vi "Parameter Filter - By Label Decimal.vi"(2 "Label Decimal":i32, 7 "Parameters Array (in)":T1[](array[typedef])) -> (8 "Filtered Parameters Array (out)":T1[](array[typedef]))   [LabVIEW 2017] (continued)
"Channel Speed"=100, "Label Decimal"=117, "Label Name"="Label_165", "Min Rate (mS)"=720, "Max Rate (mS)"=1080, "SDI"=2, "SSM"=0, "Create SDI"=FALSE, "Create SSM"=FALSE, "Create Parity"=FALSE, "Parameter Name"="eng_rb2_lbl165_b10_28", "Start Bit"=10, "Number of Bits"=19, "Scale"="1", "Offset"="0", "Signed"=FALSE, "Unit"="N/A", "Encoding"=enum."Discrete", "Default Value"="0"}, {"Core Number"=0, "Channel Number"=23, "Channel Name"="ENG_RB2", "Channel Speed"=100, "Label Decimal"=119, "Label Name"="Label_167", "Min Rate (mS)"=720, "Max Rate (mS)"=1080, "SDI"=2, "SSM"=0, "Create SDI"=FALSE, "Create SSM"=FALSE, "Create Parity"=FALSE, "Parameter Name"="eng_rb2_lbl167_b10_28", "Start Bit"=10, "Number of Bits"=19, "Scale"="1", "Offset"="0", "Signed"=FALSE, "Unit"="N/A", "Encoding"=enum."Discrete", "Default Value"="0"}, {"Core Number"=0, "Channel Number"=23, "Channel Name"="ENG_RB2", "Channel Speed"=100, "Label Decimal"=120, "Label Name"="Label_170", "Min Rate (mS)"=720, "Max Rate (mS)"=1080, "SDI"=2, "SSM"=0, "Create SDI"=FALSE, "Create SSM"=FALSE, "Create Parity"=FALSE, "Parameter Name"="eng_rb2_lbl170_b10_28", "Start Bit"=10, "Number of Bits"=19, "Scale"="1", "Offset"="0", "Signed"=FALSE, "Unit"="N/A", "Encoding"=enum."Discrete", "Default Value"="0"}, {"Core Number"=0, "Channel Number"=23, "Channel Name"="ENG_RB2", "Channel Speed"=100, "Label Decimal"=125, "Label Name"="Label_175", "Min Rate (mS)"=720, "Max Rate (mS)"=1080, "SDI"=2, "SSM"=0, "Create SDI"=FALSE, "Create SSM"=FALSE, "Create Parity"=FALSE, "Parameter Name"="eng_rb2_lbl175_b10_28", "Start Bit"=10, "Number of Bits"=19, "Scale"="1", "Offset"="0", "Signed"=FALSE, "Unit"="N/A", "Encoding"=enum."Discrete", "Default Value"="0"}, {"Core Number"=0, "Channel Number"=23, "Channel Name"="ENG_RB2", "Channel Speed"=100, "Label Decimal"=126, "Label Name"="Label_176", "Min Rate (mS)"=720, "Max Rate (mS)"=1080, "SDI"=2, "SSM"=0, "Create SDI"=FALSE, "Create SSM"=FALSE, "Create Parity"=FALSE, "Parameter Name"="eng_rb2_lbl176_b10_28", "Start Bit"=10, "Number of Bits"=19, "Scale"="1", "Offset"="0", "Signed"=FALSE, "Unit"="N/A", "Encoding"=enum."Discrete", "Default Value"="0"}, {"Core Number"=0, "Channel Number"=23, "Channel Name"="ENG_RB2", "Channel Speed"=100, "Label Decimal"=127, "Label Name"="Label_177", "Min Rate (mS)"=720, "Max Rate (mS)"=1080, "SDI"=2, "SSM"=0, "Create SDI"=FALSE, "Create SSM"=FALSE, "Create Parity"=FALSE, "Parameter Name"="eng_rb2_lbl177_b10_28", "Start Bit"=10, "Number of Bits"=19, "Scale"="1", "Offset"="0", "Signed"=FALSE, "Unit"="N/A", "Encoding"=enum."Discrete", "Default Value"="0"}, {"Core Number"=0, "Channel Number"=23, "Channel Name"="ENG_RB2", "Channel Speed"=100, "Label Decimal"=129, "Label Name"="Label_201", "Min Rate (mS)"=720, "Max Rate (mS)"=1080, "SDI"=2, "SSM"=0, "Create SDI"=FALSE, "Create SSM"=FALSE, "Create Parity"=FALSE, "Parameter Name"="eng_rb2_lbl201_b10_28", "Start Bit"=10, "Number of Bits"=19, "Scale"="1", "Offset"="0", "Signed"=FALSE, "Unit"="N/A", "Encoding"=enum."Discrete", "Default Value"="0"}, {"Core Number"=0, "Channel Number"=23, "Channel Name"="ENG_RB2", "Channel Speed"=100, "Label Decimal"=130, "Label Name"="Label_202", "Min Rate (mS)"=720, "Max Rate (mS)"=1080, "SDI"=2, "SSM"=0, "Create SDI"=FALSE, "Create SSM"=FALSE, "Create Parity"=FALSE, "Parameter Name"="eng_rb2_lbl202_b10_28", "Start Bit"=10, "Number of Bits"=19, "Scale"="1", "Offset"="0", "Signed"=FALSE, "Unit"="N/A", "Encoding"=enum."Discrete", "Default Value"="0"}, {"Core Number"=0, "Channel Number"=23, "Channel Name"="ENG_RB2", "Channel Speed"=100, "Label Decimal"=132, "Label Name"="Label_204", "Min Rate (mS)"=720, "Max Rate (mS)"=1080, "SDI"=2, "SSM"=0, "Create SDI"=FALSE, "Create SSM"=FALSE, "Create Parity"=FALSE, "Parameter Name"="eng_rb2_lbl204_b10_28", "Start Bit"=10, "Number of Bits"=19, "Scale"="1", "Offset"="0", "Signed"=FALSE, "Unit"="N/A", "Encoding"=enum."Discrete", "Default Value"="0"}, {"Core Number"=0, "Channel Number"=23, "Channel Name"="ENG_RB2", "Channel Speed"=100, "Label Decimal"=139, "Label Name"="Label_213", "Min Rate (mS)"=800, "Max Rate (mS)"=1200, "SDI"=2, "SSM"=0, "Create SDI"=FALSE, "Create SSM"=FALSE, "Create Parity"=FALSE, "Parameter Name"="eng_rb2_lbl213_b10_28", "Start Bit"=10, "Number of Bits"=19, "Scale"="1", "Offset"="0", "Signed"=FALSE, "Unit"="N/A", "Encoding"=enum."Discrete", "Default Value"="0"}, {"Core Number"=0, "Channel Number"=23, "Channel Name"="ENG_RB2", "Channel Speed"=100, "Label Decimal"=64, "Label Name"="Label_100", "Min Rate (mS)"=800, "Max Rate (mS)"=1200, "SDI"=2, "SSM"=0, "Create SDI"=FALSE, "Create SSM"=FALSE, "Create Parity"=FALSE, "Parameter Name"="eng_rb2_lbl100_b13_27", "Start Bit"=13, "Number of Bits"=15, "Scale"="1", "Offset"="0", "Signed"=FALSE, "Unit"="N/A", "Encoding"=enum."Discrete", "Default Value"="0"}, {"Core Number"=0, "Channel Number"=23, "Channel Name"="ENG_RB2", "Channel Speed"=100, "Label Decimal"=66, "Label Name"="Label_102", "Min Rate (mS)"=800, "Max Rate (mS)"=1200, "SDI"=2, "SSM"=0, "Create SDI"=FALSE, "Create SSM"=FALSE, "Create Parity"=FALSE, "Parameter Name"="eng_rb2_lbl102_b13_27", "Start Bit"=13, "Number of Bits"=15, "Scale"="1", "Offset"="0", "Signed"=FALSE, "Unit"="N/A", "Encoding"=enum."Discrete", "Default Value"="0"}, {"Core Number"=0, "Channel Number"=1, "Channel Name"="RDC20_ENG_LA1", "Channel Speed"=100, "Label Decimal"=213, "Label Name"="Label_325", "Min Rate (mS)"=40, "Max Rate (mS)"=60, "SDI"=0, "SSM"=3, "Create SDI"=FALSE, "Create SSM"=FALSE, "Create Parity"=FALSE, "Parameter Name"="rdc20_eng_la1_lbl325_b10_28", "Start Bit"=10, "Number of Bits"=19, "Scale"="0.0006866", "Offset"="0", "Signed"=TRUE, "Unit"="Degrees", "Encoding"=enum."BNR", "Default Value"="0"}, {"Core Number"=0, "Channel Number"=1, "Channel Name"="RDC20_ENG_LA1", "Channel Speed"=100, "Label Decimal"=91, "Label Name"="Label_133", "Min Rate (mS)"=40, "Max Rate (mS)"=60, "SDI"=0, "SSM"=3, "Create SDI"=FALSE, "Create SSM"=FALSE, "Create Parity"=FALSE, "Parameter Name"="rdc20_eng_la1_lbl133_b10_28", "Start Bit"=10, "Number of Bits"=19, "Scale"="0.0006866", "Offset"="0", "Signed"=TRUE, "Unit"="Degrees", "Encoding"=enum."BNR", "Default Value"="0"}, {"Core Number"=0, "Channel Number"=1, "Channel Name"="RDC20_ENG_LA1", "Channel Speed"=100, "Label Decimal"=104, "Label Name"="Label_150", "Min Rate (mS)"=800, "Max Rate (mS)"=1200, "SDI"=0, "SSM"=3, "Create SDI"=FALSE, "Create SSM"=FALSE, "Create Parity"=FALSE, "Parameter Name"="rdc20_eng_la1_lbl150_b11_27", "Start Bit"=11, "Number of Bits"=17, "Scale"="1", "Offset"="0", "Signed"=FALSE, "Unit"="hh.mm.ss", "Encoding"=enum."BNR", "Default Value"="0"}, {"Core Number"=0, "Channel Number"=1, "Channel Name"="RDC20_ENG_LA1", "Channel Speed"=100, "Label Decimal"=39, "Label Name"="Label_47", "Min Rate (mS)"=800, "Max Rate (mS)"=1200, "SDI"=0, "SSM"=3, "Create SDI"=FALSE, "Create SSM"=FALSE, "Create Parity"=FALSE, "Parameter Name"="rdc20_eng_la1_lbl47_b10_27", "Start Bit"=10, "Number of Bits"=18, "Scale"="1", "Offset"="0", "Signed"=FALSE, "Unit"="N/A", "Encoding"=enum."BNR", "Default Value"="0"}, {"Core Number"=0, "Channel Number"=1, "Channel Name"="RDC20_ENG_LA1", "Channel Speed"=100, "Label Decimal"=188, "Label Name"="Label_274", "Min Rate (mS)"=800, "Max Rate (mS)"=1200, "SDI"=0, "SSM"=3, "Create SDI"=FALSE, "Create SSM"=FALSE, "Create Parity"=FALSE, "Parameter Name"="rdc20_eng_la1_lbl274_b18_28", "Start Bit"=18, "Number of Bits"=11, "Scale"="0.5", "Offset"="0", "Signed"=TRUE, "Unit"="Deg C", "Encoding"=enum."BNR", "Default Value"="0"}, {"Core Number"=0, "Channel Number"=1, "Channel Name"="RDC20_ENG_LA1", "Channel Speed"=100, "Label Decimal"=189, "Label Name"="Label_275", "Min Rate (mS)"=800, "Max Rate (mS)"=1200, "SDI"=0, "SSM"=3, "Create SDI"=FALSE, "Create SSM"=FALSE, "Create Parity"=FALSE, "Parameter Name"="rdc20_eng_la1_lbl275_b18_28", "Start Bit"=18, "Number of Bits"=11, "Scale"="0.5", "Offset"="0", "Signed"=TRUE, "Unit"="Deg C", "Encoding"=enum."BNR", "Default Value"="0"}, {"Core Number"=0, "Channel Number"=1, "Channel Name"="RDC20_ENG_LA1", "Channel Speed"=100, "Label Decimal"=184, "Label Name"="Label_270", "Min Rate (mS)"=80, "Max Rate (mS)"=120, "SDI"=0, "SSM"=0, "Create SDI"=FALSE, "Create SSM"=FALSE, "Create Parity"=FALSE, "Parameter Name"="rdc20_eng_la1_lbl270_b10_28", "Start Bit"=10, "Number of Bits"=19, "Scale"="1", "Offset"="0", "Signed"=FALSE, "Unit"="N/A", "Encoding"=enum."Discrete", "Default Value"="0"}, {"Core Number"=0, "Channel Number"=1, "Channel Name"="RDC20_ENG_LA1", "Channel Speed"=100, "Label Decimal"=185, "Label Name"="Label_271", "Min Rate (mS)"=80, "Max Rate (mS)"=120, "SDI"=0, "SSM"=0, "Create SDI"=FALSE, "Create SSM"=FALSE, "Create Parity"=FALSE, "Parameter Name"="rdc20_eng_la1_lbl271_b10_28", "Start Bit"=10, "Number of Bits"=19, "Scale"="1", "Offset"="0", "Signed"=FALSE, "Unit"="N/A", "Encoding"=enum."Discrete", "Default Value"="0"}, {"Core Number"=0, "Channel Number"=1, "Channel Name"="RDC20_ENG_LA1", "Channel Speed"=100, "Label Decimal"=186, "Label Name"="Label_272", "Min Rate (mS)"=80, "Max Rate (mS)"=120, "SDI"=0, "SSM"=0, "Create SDI"=FALSE, "Create SSM"=FALSE, "Create Parity"=FALSE, "Parameter Name"="rdc20_eng_la1_lbl272_b10_28", "Start Bit"=10, "Number of Bits"=19, "Scale"="1", "Offset"="0", "Signed"=FALSE, "Unit"="N/A", "Encoding"=enum."Discrete", "Default Value"="0"}, {"Core Number"=0, "Channel Number"=1, "Channel Name"="RDC20_ENG_LA1", "Channel Speed"=100, "Label Decimal"=187, "Label Name"="Label_273", "Min Rate (mS)"=80, "Max Rate (mS)"=120, "SDI"=0, "SSM"=0, "Create SDI"=FALSE, "Create SSM"=FALSE, "Create Parity"=FALSE, "Parameter Name"="rdc20_eng_la1_lbl273_b10_28", "Start Bit"=10, "Number of Bits"=19, "Scale"="1", "Offset"="0", "Signed"=FALSE, "Unit"="N/A", "Encoding"=enum."Discrete", "Default Value"="0"}, {"Core Number"=0, "Channel Number"=1, "Channel Name"="RDC20_ENG_LA1", "Channel Speed"=100, "Label Decimal"=151, "Label Name"="Label_227", "Min Rate (mS)"=80, "Max Rate (mS)"=120, "SDI"=0, "SSM"=0, "Create SDI"=FALSE, "Create SSM"=FALSE, "Create Parity"=FALSE, "Parameter Name"="rdc20_eng_la1_lbl227_b10_28", "Start Bit"=10, "Number of Bits"=19, "Scale"="1", "Offset"="0", "Signed"=FALSE, "Unit"="N/A", "Encoding"=enum."Discrete", "Default Value"="0"}, {"Core Number"=0, "Channel Number"=1, "Channel Name"="RDC20_ENG_LA1", "Channel Speed"=100, "Label Decimal"=105, "Label Name"="Label_151", "Min Rate (mS)"=800, "Max Rate (mS)"=1200, "SDI"=0, "SSM"=0, "Create SDI"=FALSE, "Create SSM"=FALSE, "Create Parity"=FALSE, "Parameter Name"="rdc20_eng_la1_lbl151_b10_27", "Start Bit"=10, "Number of Bits"=18, "Scale"="1", "Offset"="0", "Signed"=FALSE, "Unit"="N/A", "Encoding"=enum."Discrete", "Default Value"="0"}, {"Core Number"=0, "Channel Number"=2, "Channel Name"="RDC20_ENG_LA2", "Channel Speed"=100, "Label Decimal"=213, "Label Name"="Label_325", "Min Rate (mS)"=40, "Max Rate (mS)"=60, "SDI"=0, "SSM"=3, "Create SDI"=FALSE, "Create SSM"=FALSE, "Create Parity"=FALSE, "Parameter Name"="rdc20_eng_la2_lbl325_b10_28", "Start Bit"=10, "Number of Bits"=19, "Scale"="0.0006866", "Offset"="0", "Signed"=TRUE, "Unit"="Degrees", "Encoding"=enum."BNR", "Default Value"="0"}, {"Core Number"=0, "Channel Number"=2, "Channel Name"="RDC20_ENG_LA2", "Channel Speed"=100, "Label Decimal"=91, "Label Name"="Label_133", "Min Rate (mS)"=40, "Max Rate (mS)"=60, "SDI"=0, "SSM"=3, "Create SDI"=FALSE, "Create SSM"=FALSE, "Create Parity"=FALSE, "Parameter Name"="rdc20_eng_la2_lbl133_b10_28", "Start Bit"=10, "Number of Bits"=19, "Scale"="0.0006866", "Offset"="0", "Signed"=TRUE, "Unit"="Degrees", "Encoding"=enum."BNR", "Default Value"="0"}, {"Core Number"=0, "Channel Number"=2, "Channel Name"="RDC20_ENG_LA2", "Channel Speed"=100, "Label Decimal"=104, "Label Name"="Label_150", "Min Rate (mS)"=800, "Max Rate (mS)"=1200, "SDI"=0, "SSM"=3, "Create SDI"=FALSE, "Create SSM"=FALSE, "Create Parity"=FALSE, "Parameter Name"="rdc20_eng_la2_lbl150_b11_27", "Start Bit"=11, "Number of Bits"=17, "Scale"="1", "Offset"="0", "Signed"=FALSE, "Unit"="hh.mm.ss", "Encoding"=enum."BNR", "Default Value"="0"}, {"Core Number"=0, "Channel Number"=2, "Channel Name"="RDC20_ENG_LA2", "Channel Speed"=100, "Label Decimal"=39, "Label Name"="Label_47", "Min Rate (mS)"=800, "Max Rate (mS)"=1200, "SDI"=0, "SSM"=3, "Create SDI"=FALSE, "Create SSM"=FALSE, "Create Parity"=FALSE, "Parameter Name"="rdc20_eng_la2_lbl47_b10_27", "Start Bit"=10, "Number of Bits"=18, "Scale"="1", "Offset"="0", "Signed"=FALSE, "Unit"="N/A", "Encoding"=enum."BNR", "Default Value"="0"}, {"Core Number"=0, "Channel Number"=2, "Channel Name"="RDC20_ENG_LA2", "Channel Speed"=100, "Label Decimal"=188, "Label Name"="Label_274", "Min Rate (mS)"=800, "Max Rate (mS)"=1200, "SDI"=0, "SSM"=3, "Create SDI"=FALSE, "Create SSM"=FALSE, "Create Parity"=FALSE, "Parameter Name"="rdc20_eng_la2_lbl274_b18_28", "Start Bit"=18, "Number of Bits"=11, "Scale"="0.5", "Offset"="0", "Signed"=TRUE, "Unit"="Deg C", "Encoding"=enum."BNR", "Default Value"="0"}, {"Core Number"=0, "Channel Number"=2, "Channel Name"="RDC20_ENG_LA2", "Channel Speed"=100, "Label Decimal"=189, "Label Name"="Label_275", "Min Rate (mS)"=800, "Max Rate (mS)"=1200, "SDI"=0, "SSM"=3, "Create SDI"=FALSE, "Create SSM"=FALSE, "Create Parity"=FALSE, "Parameter Name"="rdc20_eng_la2_lbl275_b18_28", "Start Bit"=18, "Number of Bits"=11, "Scale"="0.5", "Offset"="0", "Signed"=TRUE, "Unit"="Deg C", "Encoding"=enum."BNR", "Default Value"="0"}, {"Core Number"=0, "Channel Number"=2, "Channel Name"="RDC20_ENG_LA2", "Channel Speed"=100, "Label Decimal"=184, "Label Name"="Label_270", "Min Rate (mS)"=80, "Max Rate (mS)"=120, "SDI"=0, "SSM"=0, "Create SDI"=FALSE, "Create SSM"=FALSE, "Create Parity"=FALSE, "Parameter Name"="rdc20_eng_la2_lbl270_b10_28", "Start Bit"=10, "Number of Bits"=19, "Scale"="1", "Offset"="0", "Signed"=FALSE, "Unit"="N/A", "Encoding"=enum."Discrete", "Default Value"="0"}, {"Core Number"=0, "Channel Number"=2, "Channel Name"="RDC20_ENG_LA2", "Channel Speed"=100, "Label Decimal"=185, "Label Name"="Label_271", "Min Rate (mS)"=80, "Max Rate (mS)"=120, "SDI"=0, "SSM"=0, "Create SDI"=FALSE, "Create SSM"=FALSE, "Create Parity"=FALSE, "Parameter Name"="rdc20_eng_la2_lbl271_b10_28", "Start Bit"=10, "Number of Bits"=19, "Scale"="1", "Offset"="0", "Signed"=FALSE, "Unit"="N/A", "Encoding"=enum."Discrete", "Default Value"="0"}, {"Core Number"=0, "Channel Number"=2, "Channel Name"="RDC20_ENG_LA2", "Channel Speed"=100, "Label Decimal"=186, "Label Name"="Label_272", "Min Rate (mS)"=80, "Max Rate (mS)"=120, "SDI"=0, "SSM"=0, "Create SDI"=FALSE, "Create SSM"=FALSE, "Create Parity"=FALSE, "Parameter Name"="rdc20_eng_la2_lbl272_b10_28", "Start Bit"=10, "Number of Bits"=19, "Scale"="1", "Offset"="0", "Signed"=FALSE, "Unit"="N/A", "Encoding"=enum."Discrete", "Default Value"="0"}, {"Core Number"=0, "Channel Number"=2, "Channel Name"="RDC20_ENG_LA2", "Channel Speed"=100, "Label Decimal"=187, "Label Name"="Label_273", "Min Rate (mS)"=80, "Max Rate (mS)"=120, "SDI"=0, "SSM"=0, "Create SDI"=FALSE, "Create SSM"=FALSE, "Create Parity"=FALSE, "Parameter Name"="rdc20_eng_la2_lbl273_b10_28", "Start Bit"=10, "Number of Bits"=19, "Scale"="1", "Offset"="0", "Signed"=FALSE, "Unit"="N/A", "Encoding"=enum."Discrete", "Default Value"="0"}, {"Core Number"=0, "Channel Number"=2, "Channel Name"="RDC20_ENG_LA2", "Channel Speed"=100, "Label Decimal"=151, "Label Name"="Label_227", "Min Rate (mS)"=80, "Max Rate (mS)"=120, "SDI"=0, "SSM"=0, "Create SDI"=FALSE, "Create SSM"=FALSE, "Create Parity"=FALSE, "Parameter Name"="rdc20_eng_la2_lbl227_b10_28", "Start Bit"=10, "Number of Bits"=19, "Scale"="1", "Offset"="0", "Signed"=FALSE, "Unit"="N/A", "Encoding"=enum."Discrete", "Default Value"="0"}, {"Core Number"=0, "Channel Number"=2, "Channel Name"="RDC20_ENG_LA2", "Channel Speed"=100, "Label Decimal"=105, "Label Name"="Label_151", "Min Rate (mS)"=800, "Max Rate (mS)"=1200, "SDI"=0, "SSM"=0, "Create SDI"=FALSE, "Create SSM"=FALSE, "Create Parity"=FALSE, "Parameter Name"="rdc20_eng_la2_lbl151_b10_27", "Start Bit"=10, "Number of Bits"=18, "Scale"="1", "Offset"="0", "Signed"=FALSE, "Unit"="N/A", "Encoding"=enum."Discrete", "Default Value"="0"}, {"Core Number"=0, "Channel Number"=3, "Channel Name"="RDC17_ENG_LB1", "Channel Speed"=100, "Label Decimal"=213, "Label Name"="Label_325", "Min Rate (mS)"=40, "Max Rate (mS)"=60, "SDI"=1, "SSM"=3, "Create SDI"=FALSE, "Create SSM"=FALSE, "Create Parity"=FALSE, "Parameter Name"="rdc17_eng_lb1_lbl325_b10_28", "Start Bit"=10, "Number of Bits"=19, "Scale"="0.0006866", "Offset"="0", "Signed"=TRUE, "Unit"="Degrees", "Encoding"=enum."BNR", "Default Value"="0"}, {"Core Number"=0, "Channel Number"=3, "Channel Name"="RDC17_ENG_LB1", "Channel Speed"=100, "Label Decimal"=91, "Label Name"="Label_133", "Min Rate (mS)"=40, "Max Rate (mS)"=60, "SDI"=1, "SSM"=3, "Create SDI"=FALSE, "Create SSM"=FALSE, "Create Parity"=FALSE, "Parameter Name"="rdc17_eng_lb1_lbl133_b10_28", "Start Bit"=10, "Number of Bits"=19, "Scale"="0.0006866", "Offset"="0", "Signed"=TRUE, "Unit"="Degrees", "Encoding"=enum."BNR", "Default Value"="0"}, {"Core Number"=0, "Channel Number"=3, "Channel Name"="RDC17_ENG_LB1", "Channel Speed"=100, "Label Decimal"=104, "Label Name"="Label_150", "Min Rate (mS)"=800, "Max Rate (mS)"=1200, "SDI"=1, "SSM"=3, "Create SDI"=FALSE, "Create SSM"=FALSE, "Create Parity"=FALSE, "Parameter Name"="rdc17_eng_lb1_lbl150_b11_27", "Start Bit"=11, "Number of Bits"=17, "Scale"="1", "Offset"="0", "Signed"=FALSE, "Unit"="hh.mm.ss", "Encoding"=enum."BNR", "Default Value"="0"}, {"Core Number"=0, "Channel Number"=3, "Channel Name"="RDC17_ENG_LB1", "Channel Speed"=100, "Label Decimal"=39, "Label Name"="Label_47", "Min Rate (mS)"=800, "Max Rate (mS)"=1200, "SDI"=1, "SSM"=3, "Create SDI"=FALSE, "Create SSM"=FALSE, "Create Parity"=FALSE, "Parameter Name"="rdc17_eng_lb1_lbl47_b10_27", "Start Bit"=10, "Number of Bits"=18, "Scale"="1", "Offset"="0", "Signed"=FALSE, "Unit"="N/A", "Encoding"=enum."BNR", "Default Value"="0"}, {"Core Number"=0, "Channel Number"=3, "Channel Name"="RDC17_ENG_LB1", "Channel Speed"=100, "Label Decimal"=188, "Label Name"="Label_274", "Min Rate (mS)"=800, "Max Rate (mS)"=1200, "SDI"=1, "SSM"=3, "Create SDI"=FALSE, "Create SSM"=FALSE, "Create Parity"=FALSE, "Parameter Name"="rdc17_eng_lb1_lbl274_b18_28", "Start Bit"=18, "Number of Bits"=11, "Scale"="0.5", "Offset"="0", "Signed"=TRUE, "Unit"="Deg C", "Encoding"=enum."BNR", "Default Value"="0"}, {"Core Number"=0, "Channel Number"=3, "Channel Name"="RDC17_ENG_LB1", "Channel Speed"=100, "Label Decimal"=189, "Label Name"="Label_275", "Min Rate (mS)"=800, "Max Rate (mS)"=1200, "SDI"=1, "SSM"=3, "Create SDI"=FALSE, "Create SSM"=FALSE, "Create Parity"=FALSE, "Parameter Name"="rdc17_eng_lb1_lbl275_b18_28", "Start Bit"=18, "Number of Bits"=11, "Scale"="0.5", "Offset"="0", "Signed"=TRUE, "Unit"="Deg C", "Encoding"=enum."BNR", "Default Value"="0"}, {"Core Number"=0, "Channel Number"=3, "Channel Name"="RDC17_ENG_LB1", "Channel Speed"=100, "Label Decimal"=184, "Label Name"="Label_270", "Min Rate (mS)"=80, "Max Rate (mS)"=120, "SDI"=1, "SSM"=0, "Create SDI"=FALSE, "Create SSM"=FALSE, "Create Parity"=FALSE, "Parameter Name"="rdc17_eng_lb1_lbl270_b10_28", "Start Bit"=10, "Number of Bits"=19, "Scale"="1", "Offset"="0", "Signed"=FALSE, "Unit"="N/A", "Encoding"=enum."Discrete", "Default Value"="0"}, {"Core Number"=0, "Channel Number"=3, "Channel Name"="RDC17_ENG_LB1", "Channel Speed"=100, "Label Decimal"=185, "Label Name"="Label_271", "Min Rate (mS)"=80, "Max Rate (mS)"=120, "SDI"=1, "SSM"=0, "Create SDI"=FALSE, "Create SSM"=FALSE, "Create Parity"=FALSE, "Parameter Name"="rdc17_eng_lb1_lbl271_b10_28", "Start Bit"=10, "Number of Bits"=19, "Scale"="1", "Offset"="0", "Signed"=FALSE, "Unit"="N/A", "Encoding"=enum."Discrete", "Default Value"="0"}, {"Core Number"=0, "Channel Number"=3, "Channel Name"="RDC17_ENG_LB1", "Channel Speed"=100, "Label Decimal"=186, "Label Name"="Label_272", "Min Rate (mS)"=80, "Max Rate (mS)"=120, "SDI"=1, "SSM"=0, "Create SDI"=FALSE, "Create SSM"=FALSE, "Create Parity"=FALSE, "Parameter Name"="rdc17_eng_lb1_lbl272_b10_28", "Start Bit"=10, "Number of Bits"=19, "Scale"="1", "Offset"="0", "Signed"=FALSE, "Unit"="N/A", "Encoding"=enum."Discrete", "Default Value"="0"}, {"Core Number"=0, "Channel Number"=3, "Channel Name"="RDC17_ENG_LB1", "Channel Speed"=100, "Label Decimal"=187, "Label Name"="Label_273", "Min Rate (mS)"=80, "Max Rate (mS)"=120, "SDI"=1, "SSM"=0, "Create SDI"=FALSE, "Create SSM"=FALSE, "Create Parity"=FALSE, "Parameter Name"="rdc17_eng_lb1_lbl273_b10_28", "Start Bit"=10, "Number of Bits"=19, "Scale"="1", "Offset"="0", "Signed"=FALSE, "Unit"="N/A", "Encoding"=enum."Discrete", "Default Value"="0"}, {"Core Number"=0, "Channel Number"=3, "Channel Name"="RDC17_ENG_LB1", "Channel Speed"=100, "Label Decimal"=151, "Label Name"="Label_227", "Min Rate (mS)"=80, "Max Rate (mS)"=120, "SDI"=1, "SSM"=0, "Create SDI"=FALSE, "Create SSM"=FALSE, "Create Parity"=FALSE, "Parameter Name"="rdc17_eng_lb1_lbl227_b10_28", "Start Bit"=10, "Number of Bits"=19, "Scale"="1", "Offset"="0", "Signed"=FALSE, "Unit"="N/A", "Encoding"=enum."Discrete", "Default Value"="0"}, {"Core Number"=0, "Channel Number"=3, "Channel Name"="RDC17_ENG_LB1", "Channel Speed"=100, "Label Decimal"=105, "Label Name"="Label_151", "Min Rate (mS)"=800, "Max Rate (mS)"=1200, "SDI"=1, "SSM"=0, "Create SDI"=FALSE, "Create SSM"=FALSE, "Create Parity"=FALSE, "Parameter Name"="rdc17_eng_lb1_lbl151_b10_27", "Start Bit"=10, "Number of Bits"=18, "Scale"="1", "Offset"="0", "Signed"=FALSE, "Unit"="N/A", "Encoding"=enum."Discrete", "Default Value"="0"}, {"Core Number"=0, "Channel Number"=4, "Channel Name"="RDC17_ENG_LB2", "Channel Speed"=100, "Label Decimal"=213, "Label Name"="Label_325", "Min Rate (mS)"=40, "Max Rate (mS)"=60, "SDI"=1, "SSM"=3, "Create SDI"=FALSE, "Create SSM"=FALSE, "Create Parity"=FALSE, "Parameter Name"="rdc17_eng_lb2_lbl325_b10_28", "Start Bit"=10, "Number of Bits"=19, "Scale"="0.0006866", "Offset"="0", "Signed"=TRUE, "Unit"="Degrees", "Encoding"=enum."BNR", "Default Value"="0"}, {"Core Number"=0, "Channel Number"=4, "Channel Name"="RDC17_ENG_LB2", "Channel Speed"=100, "Label Decimal"=91, "Label Name"="Label_133", "Min Rate (mS)"=40, "Max Rate (mS)"=60, "SDI"=1, "SSM"=3, "Create SDI"=FALSE, "Create SSM"=FALSE, "Create Parity"=FALSE, "Parameter Name"="rdc17_eng_lb2_lbl133_b10_28", "Start Bit"=10, "Number of Bits"=19, "Scale"="0.0006866", "Offset"="0", "Signed"=TRUE, "Unit"="Degrees", "Encoding"=enum."BNR", "Default Value"="0"}, {"Core Number"=0, "Channel Number"=4, "Channel Name"="RDC17_ENG_LB2", "Channel Speed"=100, "Label Decimal"=104, "Label Name"="Label_150", "Min Rate (mS)"=800, "Max Rate (mS)"=1200, "SDI"=1, "SSM"=3, "Create SDI"=FALSE, "Create SSM"=FALSE, "Create Parity"=FALSE, "Parameter Name"="rdc17_eng_lb2_lbl150_b11_27", "Start Bit"=11, "Number of Bits"=17, "Scale"="1", "Offset"="0", "Signed"=FALSE, "Unit"="hh.mm.ss", "Encoding"=enum."BNR", "Default Value"="0"}, {"Core Number"=0, "Channel Number"=4, "Channel Name"="RDC17_ENG_LB2", "Channel Speed"=100, "Label Decimal"=39, "Label Name"="Label_47", "Min Rate (mS)"=800, "Max Rate (mS)"=1200, "SDI"=1, "SSM"=3, "Create SDI"=FALSE, "Create SSM"=FALSE, "Create Parity"=FALSE, "Parameter Name"="rdc17_eng_lb2_lbl47_b10_27", "Start Bit"=10, "Number of Bits"=18, "Scale"="1", "Offset"="0", "Signed"=FALSE, "Unit"="N/A", "Encoding"=enum."BNR", "Default Value"="0"}, {"Core Number"=0, "Channel Number"=4, "Channel Name"="RDC17_ENG_LB2", "Channel Speed"=100, "Label Decimal"=188, "Label Name"="Label_274", "Min Rate (mS)"=800, "Max Rate (mS)"=1200, "SDI"=1, "SSM"=3, "Create SDI"=FALSE, "Create SSM"=FALSE, "Create Parity"=FALSE, "Parameter Name"="rdc17_eng_lb2_lbl274_b18_28", "Start Bit"=18, "Number of Bits"=11, "Scale"="0.5", "Offset"="0", "Signed"=TRUE, "Unit"="Deg C", "Encoding"=enum."BNR", "Default Value"="0"}, {"Core Number"=0, "Channel Number"=4, "Channel Name"="RDC17_ENG_LB2", "Channel Speed"=100, "Label Decimal"=189, "Label Name"="Label_275", "Min Rate (mS)"=800, "Max Rate (mS)"=1200, "SDI"=1, "SSM"=3, "Create SDI"=FALSE, "Create SSM"=FALSE, "Create Parity"=FALSE, "Parameter Name"="rdc17_eng_lb2_lbl275_b18_28", "Start Bit"=18, "Number of Bits"=11, "Scale"="0.5", "Offset"="0", "Signed"=TRUE, "Unit"="Deg C", "Encoding"=enum."BNR", "Default Value"="0"}, {"Core Number"=0, "Channel Number"=4, "Channel Name"="RDC17_ENG_LB2", "Channel Speed"=100, "Label Decimal"=184, "Label Name"="Label_270", "Min Rate (mS)"=80, "Max Rate (mS)"=120, "SDI"=1, "SSM"=0, "Create SDI"=FALSE, "Create SSM"=FALSE, "Create Parity"=FALSE, "Parameter Name"="rdc17_eng_lb2_lbl270_b10_28", "Start Bit"=10, "Number of Bits"=19, "Scale"="1", "Offset"="0", "Signed"=FALSE, "Unit"="N/A", "Encoding"=enum."Discrete", "Default Value"="0"}, {"Core Number"=0, "Channel Number"=4, "Channel Name"="RDC17_ENG_LB2", "Channel Speed"=100, "Label Decimal"=185, "Label Name"="Label_271", "Min Rate (mS)"=80, "Max Rate (mS)"=120, "SDI"=1, "SSM"=0, "Create SDI"=FALSE, "Create SSM"=FALSE, "Create Parity"=FALSE, "Parameter Name"="rdc17_eng_lb2_lbl271_b10_28", "Start Bit"=10, "Number of Bits"=19, "Scale"="1", "Offset"="0", "Signed"=FALSE, "Unit"="N/A", "Encoding"=enum."Discrete", "Default Value"="0"}, {"Core Number"=0, "Channel Number"=4, "Channel Name"="RDC17_ENG_LB2", "Channel Speed"=100, "Label Decimal"=186, "Label Name"="Label_272", "Min Rate (mS)"=80, "Max Rate (mS)"=120, "SDI"=1, "SSM"=0, "Create SDI"=FALSE, "Create SSM"=FALSE, "Create Parity"=FALSE, "Parameter Name"="rdc17_eng_lb2_lbl272_b10_28", "Start Bit"=10, "Number of Bits"=19, "Scale"="1", "Offset"="0", "Signed"=FALSE, "Unit"="N/A", "Encoding"=enum."Discrete", "Default Value"="0"}, {"Core Number"=0, "Channel Number"=4, "Channel Name"="RDC17_ENG_LB2", "Channel Speed"=100, "Label Decimal"=187, "Label Name"="Label_273", "Min Rate (mS)"=80, "Max Rate (mS)"=120, "SDI"=1, "SSM"=0, "Create SDI"=FALSE, "Create SSM"=FALSE, "Create Parity"=FALSE, "Parameter Name"="rdc17_eng_lb2_lbl273_b10_28", "Start Bit"=10, "Number of Bits"=19, "Scale"="1", "Offset"="0", "Signed"=FALSE, "Unit"="N/A", "Encoding"=enum."Discrete", "Default Value"="0"}, {"Core Number"=0, "Channel Number"=4, "Channel Name"="RDC17_ENG_LB2", "Channel Speed"=100, "Label Decimal"=151, "Label Name"="Label_227", "Min Rate (mS)"=80, "Max Rate (mS)"=120, "SDI"=1, "SSM"=0, "Create SDI"=FALSE, "Create SSM"=FALSE, "Create Parity"=FALSE, "Parameter Name"="rdc17_eng_lb2_lbl227_b10_28", "Start Bit"=10, "Number of Bits"=19, "Scale"="1", "Offset"="0", "Signed"=FALSE, "Unit"="N/A", "Encoding"=enum."Discrete", "Default Value"="0"}, {"Core Number"=0, "Channel Number"=4, "Channel Name"="RDC17_ENG_LB2", "Channel Speed"=100, "Label Decimal"=105, "Label Name"="Label_151", "Min Rate (mS)"=800, "Max Rate (mS)"=1200, "SDI"=1, "SSM"=0, "Create SDI"=FALSE, "Create SSM"=FALSE, "Create Parity"=FALSE, "Parameter Name"="rdc17_eng_lb2_lbl151_b10_27", "Start Bit"=10, "Number of Bits"=18, "Scale"="1", "Offset"="0", "Signed"=FALSE, "Unit"="N/A", "Encoding"=enum."Discrete", "Default Value"="0"}, {"Core Number"=0, "Channel Number"=5, "Channel Name"="RDC22_ENG_RA1", "Channel Speed"=100, "Label Decimal"=213, "Label Name"="Label_325", "Min Rate (mS)"=40, "Max Rate (mS)"=60, "SDI"=2, "SSM"=3, "Create SDI"=FALSE, "Create SSM"=FALSE, "Create Parity"=FALSE, "Parameter Name"="rdc22_eng_ra1_lbl325_b10_28", "Start Bit"=10, "Number of Bits"=19, "Scale"="0.0006866", "Offset"="0", "Signed"=TRUE, "Unit"="Degrees", "Encoding"=enum."BNR", "Default Value"="0"}, {"Core Number"=0, "Channel Number"=5, "Channel Name"="RDC22_ENG_RA1", "Channel Speed"=100, "Label Decimal"=91, "Label Name"="Label_133", "Min Rate (mS)"=40, "Max Rate (mS)"=60, "SDI"=2, "SSM"=3, "Create SDI"=FALSE, "Create SSM"=FALSE, "Create Parity"=FALSE, "Parameter Name"="rdc22_eng_ra1_lbl133_b10_28", "Start Bit"=10, "Number of Bits"=19, "Scale"="0.0006866", "Offset"="0", "Signed"=TRUE, "Unit"="Degrees", "Encoding"=enum."BNR", "Default Value"="0"}, {"Core Number"=0, "Channel Number"=5, "Channel Name"="RDC22_ENG_RA1", "Channel Speed"=100, "Label Decimal"=104, "Label Name"="Label_150", "Min Rate (mS)"=800, "Max Rate (mS)"=1200, "SDI"=2, "SSM"=3, "Create SDI"=FALSE, "Create SSM"=FALSE, "Create Parity"=FALSE, "Parameter Name"="rdc22_eng_ra1_lbl150_b11_27", "Start Bit"=11, "Number of Bits"=17, "Scale"="1", "Offset"="0", "Signed"=FALSE, "Unit"="hh.mm.ss", "Encoding"=enum."BNR", "Default Value"="0"}, {"Core Number"=0, "Channel Number"=5, "Channel Name"="RDC22_ENG_RA1", "Channel Speed"=100, "Label Decimal"=39, "Label Name"="Label_47", "Min Rate (mS)"=800, "Max Rate (mS)"=1200, "SDI"=2, "SSM"=3, "Create SDI"=FALSE, "Create SSM"=FALSE, "Create Parity"=FALSE, "Parameter Name"="rdc22_eng_ra1_lbl47_b10_27", "Start Bit"=10, "Number of Bits"=18, "Scale"="1", "Offset"="0", "Signed"=FALSE, "Unit"="N/A", "Encoding"=enum."BNR", "Default Value"="0"}, {"Core Number"=0, "Channel Number"=5, "Channel Name"="RDC22_ENG_RA1", "Channel Speed"=100, "Label Decimal"=188, "Label Name"="Label_274", "Min Rate (mS)"=800, "Max Rate (mS)"=1200, "SDI"=2, "SSM"=3, "Create SDI"=FALSE, "Create SSM"=FALSE, "Create Parity"=FALSE, "Parameter Name"="rdc22_eng_ra1_lbl274_b18_28", "Start Bit"=18, "Number of Bits"=11, "Scale"="0.5", "Offset"="0", "Signed"=TRUE, "Unit"="Deg C", "Encoding"=enum."BNR", "Default Value"="0"}, {"Core Number"=0, "Channel Number"=5, "Channel Name"="RDC22_ENG_RA1", "Channel Speed"=100, "Label Decimal"=189, "Label Name"="Label_275", "Min Rate (mS)"=800, "Max Rate (mS)"=1200, "SDI"=2, "SSM"=3, "Create SDI"=FALSE, "Create SSM"=FALSE, "Create Parity"=FALSE, "Parameter Name"="rdc22_eng_ra1_lbl275_b18_28", "Start Bit"=18, "Number of Bits"=11, "Scale"="0.5", "Offset"="0", "Signed"=TRUE, "Unit"="Deg C", "Encoding"=enum."BNR", "Default Value"="0"}, {"Core Number"=0, "Channel Number"=5, "Channel Name"="RDC22_ENG_RA1", "Channel Speed"=100, "Label Decimal"=184, "Label Name"="Label_270", "Min Rate (mS)"=80, "Max Rate (mS)"=120, "SDI"=2, "SSM"=0, "Create SDI"=FALSE, "Create SSM"=FALSE, "Create Parity"=FALSE, "Parameter Name"="rdc22_eng_ra1_lbl270_b10_28", "Start Bit"=10, "Number of Bits"=19, "Scale"="1", "Offset"="0", "Signed"=FALSE, "Unit"="N/A", "Encoding"=enum."Discrete", "Default Value"="0"}, {"Core Number"=0, "Channel Number"=5, "Channel Name"="RDC22_ENG_RA1", "Channel Speed"=100, "Label Decimal"=185, "Label Name"="Label_271", "Min Rate (mS)"=80, "Max Rate (mS)"=120, "SDI"=2, "SSM"=0, "Create SDI"=FALSE, "Create SSM"=FALSE, "Create Parity"=FALSE, "Parameter Name"="rdc22_eng_ra1_lbl271_b10_28", "Start Bit"=10, "Number of Bits"=19, "Scale"="1", "Offset"="0", "Signed"=FALSE, "Unit"="N/A", "Encoding"=enum."Discrete", "Default Value"="0"}, {"Core Number"=0, "Channel Number"=5, "Channel Name"="RDC22_ENG_RA1", "Channel Speed"=100, "Label Decimal"=186, "Label Name"="Label_272", "Min Rate (mS)"=80, "Max Rate (mS)"=120, "SDI"=2, "SSM"=0, "Create SDI"=FALSE, "Create SSM"=FALSE, "Create Parity"=FALSE, "Parameter Name"="rdc22_eng_ra1_lbl272_b10_28", "Start Bit"=10, "Number of Bits"=19, "Scale"="1", "Offset"="0", "Signed"=FALSE, "Unit"="N/A", "Encoding"=enum."Discrete", "Default Value"="0"}, {"Core Number"=0, "Channel Number"=5, "Channel Name"="RDC22_ENG_RA1", "Channel Speed"=100, "Label Decimal"=187, "Label Name"="Label_273", "Min Rate (mS)"=80, "Max Rate (mS)"=120, "SDI"=2, "SSM"=0, "Create SDI"=FALSE, "Create SSM"=FALSE, "Create Parity"=FALSE, "Parameter Name"="rdc22_eng_ra1_lbl273_b10_28", "Start Bit"=10, "Number of Bits"=19, "Scale"="1", "Offset"="0", "Signed"=FALSE, "Unit"="N/A", "Encoding"=enum."Discrete", "Default Value"="0"}, {"Core Number"=0, "Channel Number"=5, "Channel Name"="RDC22_ENG_RA1", "Channel Speed"=100, "Label Decimal"=151, "Label Name"="Label_227", "Min Rate (mS)"=80, "Max Rate (mS)"=120, "SDI"=2, "SSM"=0, "Create SDI"=FALSE, "Create SSM"=FALSE, "Create Parity"=FALSE, "Parameter Name"="rdc22_eng_ra1_lbl227_b10_28", "Start Bit"=10, "Number of Bits"=19, "Scale"="1", "Offset"="0", "Signed"=FALSE, "Unit"="N/A", "Encoding"=enum."Discrete", "Default Value"="0"}, {"Core Number"=0, "Channel Number"=5, "Channel Name"="RDC22_ENG_RA1", "Channel Speed"=100, "Label Decimal"=105, "Label Name"="Label_151", "Min Rate (mS)"=800, "Max Rate (mS)"=1200, "SDI"=2, "SSM"=0, "Create SDI"=FALSE, "Create SSM"=FALSE, "Create Parity"=FALSE, "Parameter Name"="rdc22_eng_ra1_lbl151_b10_27", "Start Bit"=10, "Number of Bits"=18, "Scale"="1", "Offset"="0", "Signed"=FALSE, "Unit"="N/A", "Encoding"=enum."Discrete", "Default Value"="0"}, {"Core Number"=0, "Channel Number"=6, "Channel Name"="RDC22_ENG_RA2", "Channel Speed"=100, "Label Decimal"=213, "Label Name"="Label_325", "Min Rate (mS)"=40, "Max Rate (mS)"=60, "SDI"=2, "SSM"=3, "Create SDI"=FALSE, "Create SSM"=FALSE, "Create Parity"=FALSE, "Parameter Name"="rdc22_eng_ra2_lbl325_b10_28", "Start Bit"=10, "Number of Bits"=19, "Scale"="0.0006866", "Offset"="0", "Signed"=TRUE, "Unit"="Degrees", "Encoding"=enum."BNR", "Default Value"="0"}, {"Core Number"=0, "Channel Number"=6, "Channel Name"="RDC22_ENG_RA2", "Channel Speed"=100, "Label Decimal"=91, "Label Name"="Label_133", "Min Rate (mS)"=40, "Max Rate (mS)"=60, "SDI"=2, "SSM"=3, "Create SDI"=FALSE, "Create SSM"=FALSE, "Create Parity"=FALSE, "Parameter Name"="rdc22_eng_ra2_lbl133_b10_28", "Start Bit"=10, "Number of Bits"=19, "Scale"="0.0006866", "Offset"="0", "Signed"=TRUE, "Unit"="Degrees", "Encoding"=enum."BNR", "Default Value"="0"}, {"Core Number"=0, "Channel Number"=6, "Channel Name"="RDC22_ENG_RA2", "Channel Speed"=100, "Label Decimal"=104, "Label Name"="Label_150", "Min Rate (mS)"=800, "Max Rate (mS)"=1200, "SDI"=2, "SSM"=3, "Create SDI"=FALSE, "Create SSM"=FALSE, "Create Parity"=FALSE, "Parameter Name"="rdc22_eng_ra2_lbl150_b11_27", "Start Bit"=11, "Number of Bits"=17, "Scale"="1", "Offset"="0", "Signed"=FALSE, "Unit"="hh.mm.ss", "Encoding"=enum."BNR", "Default Value"="0"}, {"Core Number"=0, "Channel Number"=6, "Channel Name"="RDC22_ENG_RA2", "Channel Speed"=100, "Label Decimal"=39, "Label Name"="Label_47", "Min Rate (mS)"=800, "Max Rate (mS)"=1200, "SDI"=2, "SSM"=3, "Create SDI"=FALSE, "Create SSM"=FALSE, "Create Parity"=FALSE, "Parameter Name"="rdc22_eng_ra2_lbl47_b10_27", "Start Bit"=10, "Number of Bits"=18, "Scale"="1", "Offset"="0", "Signed"=FALSE, "Unit"="N/A", "Encoding"=enum."BNR", "Default Value"="0"}, {"Core Number"=0, "Channel Number"=6, "Channel Name"="RDC22_ENG_RA2", "Channel Speed"=100, "Label Decimal"=188, "Label Name"="Label_274", "Min Rate (mS)"=800, "Max Rate (mS)"=1200, "SDI"=2, "SSM"=3, "Create SDI"=FALSE, "Create SSM"=FALSE, "Create Parity"=FALSE, "Parameter Name"="rdc22_eng_ra2_lbl274_b18_28", "Start Bit"=18, "Number of Bits"=11, "Scale"="0.5", "Offset"="0", "Signed"=TRUE, "Unit"="Deg C", "Encoding"=enum."BNR", "Default Value"="0"}, {"Core Number"=0, "Channel Number"=6, "Channel Name"="RDC22_ENG_RA2", "Channel Speed"=100, "Label Decimal"=189, "Label Name"="Label_275", "Min Rate (mS)"=800, "Max Rate (mS)"=1200, "SDI"=2, "SSM"=3, "Create SDI"=FALSE, "Create SSM"=FALSE, "Create Parity"=FALSE, "Parameter Name"="rdc22_eng_ra2_lbl275_b18_28", "Start Bit"=18, "Number of Bits"=11, "Scale"="0.5", "Offset"="0", "Signed"=TRUE, "Unit"="Deg C", "Encoding"=enum."BNR", "Default Value"="0"}, {"Core Number"=0, "Channel Number"=6, "Channel Name"="RDC22_ENG_RA2", "Channel Speed"=100, "Label Decimal"=184, "Label Name"="Label_270", "Min Rate (mS)"=80, "Max Rate (mS)"=120, "SDI"=2, "SSM"=0, "Create SDI"=FALSE, "Create SSM"=FALSE, "Create Parity"=FALSE, "Parameter Name"="rdc22_eng_ra2_lbl270_b10_28", "Start Bit"=10, "Number of Bits"=19, "Scale"="1", "Offset"="0", "Signed"=FALSE, "Unit"="N/A", "Encoding"=enum."Discrete", "Default Value"="0"}, {"Core Number"=0, "Channel Number"=6, "Channel Name"="RDC22_ENG_RA2", "Channel Speed"=100, "Label Decimal"=185, "Label Name"="Label_271", "Min Rate (mS)"=80, "Max Rate (mS)"=120, "SDI"=2, "SSM"=0, "Create SDI"=FALSE, "Create SSM"=FALSE, "Create Parity"=FALSE, "Parameter Name"="rdc22_eng_ra2_lbl271_b10_28", "Start Bit"=10, "Number of Bits"=19, "Scale"="1", "Offset"="0", "Signed"=FALSE, "Unit"="N/A", "Encoding"=enum."Discrete", "Default Value"="0"}, {"Core Number"=0, "Channel Number"=6, "Channel Name"="RDC22_ENG_RA2", "Channel Speed"=100, "Label Decimal"=186, "Label Name"="Label_272", "Min Rate (mS)"=80, "Max Rate (mS)"=120, "SDI"=2, "SSM"=0, "Create SDI"=FALSE, "Create SSM"=FALSE, "Create Parity"=FALSE, "Parameter Name"="rdc22_eng_ra2_lbl272_b10_28", "Start Bit"=10, "Number of Bits"=19, "Scale"="1", "Offset"="0", "Signed"=FALSE, "Unit"="N/A", "Encoding"=enum."Discrete", "Default Value"="0"}, {"Core Number"=0, "Channel Number"=6, "Channel Name"="RDC22_ENG_RA2", "Channel Speed"=100, "Label Decimal"=187, "Label Name"="Label_273", "Min Rate (mS)"=80, "Max Rate (mS)"=120, "SDI"=2, "SSM"=0, "Create SDI"=FALSE, "Create SSM"=FALSE, "Create Parity"=FALSE, "Parameter Name"="rdc22_eng_ra2_lbl273_b10_28", "Start Bit"=10, "Number of Bits"=19, "Scale"="1", "Offset"="0", "Signed"=FALSE, "Unit"="N/A", "Encoding"=enum."Discrete", "Default Value"="0"}, {"Core Number"=0, "Channel Number"=6, "Channel Name"="RDC22_ENG_RA2", "Channel Speed"=100, "Label Decimal"=151, "Label Name"="Label_227", "Min Rate (mS)"=80, "Max Rate (mS)"=120, "SDI"=2, "SSM"=0, "Create SDI"=FALSE, "Create SSM"=FALSE, "Create Parity"=FALSE, "Parameter Name"="rdc22_eng_ra2_lbl227_b10_28", "Start Bit"=10, "Number of Bits"=19, "Scale"="1", "Offset"="0", "Signed"=FALSE, "Unit"="N/A", "Encoding"=enum."Discrete", "Default Value"="0"}, {"Core Number"=0, "Channel Number"=6, "Channel Name"="RDC22_ENG_RA2", "Channel Speed"=100, "Label Decimal"=105, "Label Name"="Label_151", "Min Rate (mS)"=800, "Max Rate (mS)"=1200, "SDI"=2, "SSM"=0, "Create SDI"=FALSE, "Create SSM"=FALSE, "Create Parity"=FALSE, "Parameter Name"="rdc22_eng_ra2_lbl151_b10_27", "Start Bit"=10, "Number of Bits"=18, "Scale"="1", "Offset"="0", "Signed"=FALSE, "Unit"="N/A", "Encoding"=enum."Discrete", "Default Value"="0"}, {"Core Number"=0, "Channel Number"=7, "Channel Name"="RDC18_ENG_RB1", "Channel Speed"=100, "Label Decimal"=213, "Label Name"="Label_325", "Min Rate (mS)"=40, "Max Rate (mS)"=60, "SDI"=3, "SSM"=3, "Create SDI"=FALSE, "Create SSM"=FALSE, "Create Parity"=FALSE, "Parameter Name"="rdc18_eng_rb1_lbl325_b10_28", "Start Bit"=10, "Number of Bits"=19, "Scale"="0.0006866", "Offset"="0", "Signed"=TRUE, "Unit"="Degrees", "Encoding"=enum."BNR", "Default Value"="0"}, {"Core Number"=0, "Channel Number"=7, "Channel Name"="RDC18_ENG_RB1", "Channel Speed"=100, "Label Decimal"=91, "Label Name"="Label_133", "Min Rate (mS)"=40, "Max Rate (mS)"=60, "SDI"=3, "SSM"=3, "Create SDI"=FALSE, "Create SSM"=FALSE, "Create Parity"=FALSE, "Parameter Name"="rdc18_eng_rb1_lbl133_b10_28", "Start Bit"=10, "Number of Bits"=19, "Scale"="0.0006866", "Offset"="0", "Signed"=TRUE, "Unit"="Degrees", "Encoding"=enum."BNR", "Default Value"="0"}, {"Core Number"=0, "Channel Number"=7, "Channel Name"="RDC18_ENG_RB1", "Channel Speed"=100, "Label Decimal"=104, "Label Name"="Label_150", "Min Rate (mS)"=800, "Max Rate (mS)"=1200, "SDI"=3, "SSM"=3, "Create SDI"=FALSE, "Create SSM"=FALSE, "Create Parity"=FALSE, "Parameter Name"="rdc18_eng_rb1_lbl150_b11_27", "Start Bit"=11, "Number of Bits"=17, "Scale"="1", "Offset"="0", "Signed"=FALSE, "Unit"="hh.mm.ss", "Encoding"=enum."BNR", "Default Value"="0"}, {"Core Number"=0, "Channel Number"=7, "Channel Name"="RDC18_ENG_RB1", "Channel Speed"=100, "Label Decimal"=39, "Label Name"="Label_47", "Min Rate (mS)"=800, "Max Rate (mS)"=1200, "SDI"=3, "SSM"=3, "Create SDI"=FALSE, "Create SSM"=FALSE, "Create Parity"=FALSE, "Parameter Name"="rdc18_eng_rb1_lbl47_b10_27", "Start Bit"=10, "Number of Bits"=18, "Scale"="1", "Offset"="0", "Signed"=FALSE, "Unit"="N/A", "Encoding"=enum."BNR", "Default Value"="0"}, {"Core Number"=0, "Channel Number"=7, "Channel Name"="RDC18_ENG_RB1", "Channel Speed"=100, "Label Decimal"=188, "Label Name"="Label_274", "Min Rate (mS)"=800, "Max Rate (mS)"=1200, "SDI"=3, "SSM"=3, "Create SDI"=FALSE, "Create SSM"=FALSE, "Create Parity"=FALSE, "Parameter Name"="rdc18_eng_rb1_lbl274_b18_28", "Start Bit"=18, "Number of Bits"=11, 
